vi "Example Callback.vi"() -> ()   [LabVIEW 2013]
uses:
  C:/tf/play/labview/Tinkerforge.dll
  Tinkerforge.dll
panel:
  in  "stop":bool
  in  "uid":string="63oL6P"
  in  "port":i32=4223
  in  "host":string="localhost"
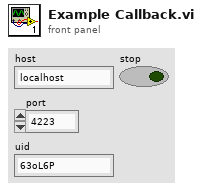
[diagram p1: front panel]
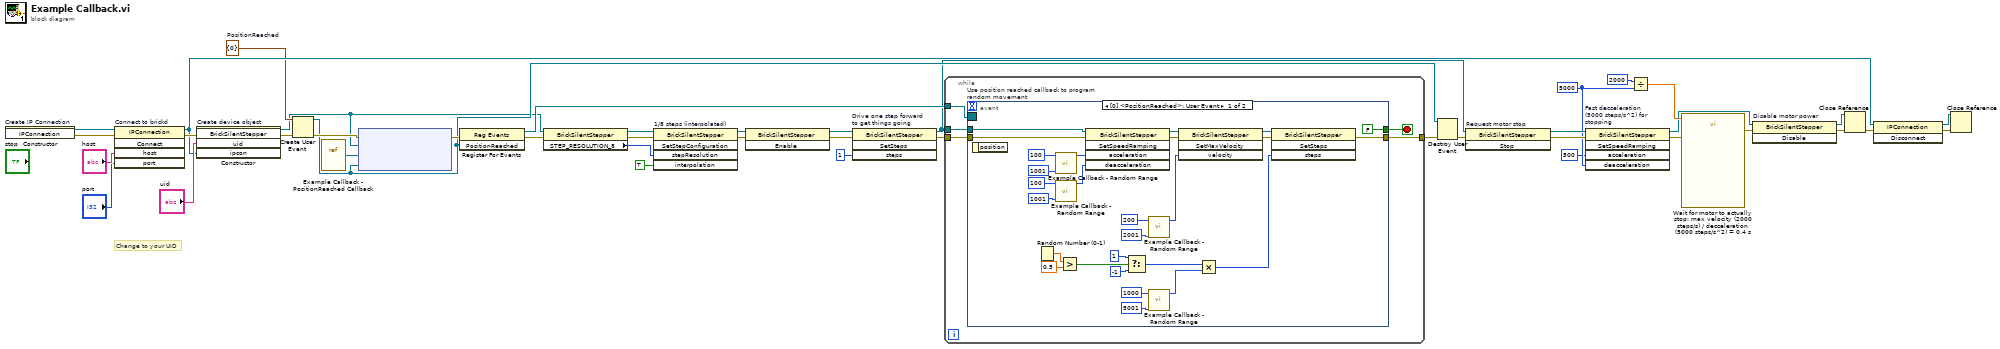
[diagram p0: block diagram]
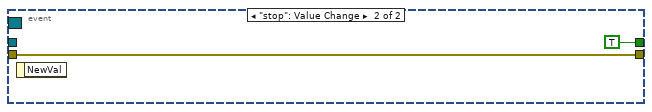
[diagram p2: hidden frame]
diagram:
  w7 = 5000 ("deacceleration")
  w29 = cluster{"position":i32} {"position"=0}  # PositionReached
  # "Change to your UID"
  n1 = constructor on="Create IP Connection" class="IPConnection"() -> (reference out=w43:refnum<k24>, error out=w23:errorcluster)  [unwired: 3 in, 1 out]
  n2 = invoke on="Connect to brickd" class="IPConnection" method="Connect"(reference=w43, error in=w23, "host"="host", "port"="port") -> (reference out=w36:refnum<k24>, error out=w39:errorcluster)  [unwired: 1 in, 3 out]
  n3 = constructor on="Create device object" class="BrickSilentStepper"(error in=w39, "uid"="uid", "ipcon"=w36) -> (reference out=w19:refnum<k24>, error out=w28:errorcluster)  [unwired: 2 in, 3 out]
  n4 = Create User Event(user event datatype=w29, error in=w28) -> (user event=w30:refnum<user-event>, error out=w34:errorcluster)
  n5 = vi-ref "Example Callback - PositionReached Callback.vi"() -> ("vi reference"=w22:refnum<vi>)
  n6 = node ("Register Event Callback")(w34, w19, w22, w30) -> (w33:errorcluster)  [unwired: 1 in, 1 out]
  n7 = register-events(error in=w33, w30) -> (reference out=w32:refnum<event-registration>, error out=w16:errorcluster)  [unwired: 1 in]
  n8 = property class="BrickSilentStepper"(reference=w19, error in=w16) -> (reference out=w18:refnum<k24>, error out=w17:errorcluster, "STEP_RESOLUTION_8"=w15:u8)
  n9 = invoke on="1/8 steps (interpolated)" class="BrickSilentStepper" method="SetStepConfiguration"(reference=w18, error in=w17, "stepResolution"=w15, "interpolation"=TRUE) -> (reference out=w20:refnum<k24>, error out=w21:errorcluster)  [unwired: 1 in, 3 out]
  n10 = invoke class="BrickSilentStepper" method="Enable"(reference=w20, error in=w21) -> (reference out=w27:refnum<k24>, error out=w26:errorcluster)  [unwired: 1 in, 1 out]
  n11 = invoke on="Drive one step forward\nto get things going" class="BrickSilentStepper" method="SetSteps"(reference=w27, error in=w26, "steps"=1) -> (reference out=w4:refnum<k24>, error out=w25:errorcluster)  [unwired: 1 in, 2 out]
  n12 = while {
    tunnel: w32 -> [w48]
    tunnel: [w47] -> w31
    tunnel: w25 -> [w46]
    tunnel: w4 -> [w45]
    stop <- w44 stop-if-true
    n13 = event "Use position reached callback to program random movement" shown="[0] <PositionReached>: User Event" {
      selector: w48 -> [_ _]
      dyn-events: _ -> [_ _]
      timeout: _ -> [_ _]
      tunnel: [w75 w76] -> w47
      tunnel: w46 -> [w71 w76]
      tunnel: w45 -> [w50 _]
      tunnel: [FALSE TRUE] -> w44
      event User Event {
        n14 = event-data() -> ()  [unwired: 1 in, 1 out]
        n15 = Random Number (0-1)() -> (number: 0 to 1=w58:dbl)
        n16 = call "Example Callback - Random Range.vi"("max"=1001, "min"=100) -> ("random"=w69:i32)  [unwired: 9 in]
        n17 = call "Example Callback - Random Range.vi"("max"=1001, "min"=100) -> ("random"=w68:i32)  [unwired: 9 in]
        n18 = Greater?(x=w58, y=0.5) -> (0:w56:bool)
        n19 = invoke class="BrickSilentStepper" method="SetSpeedRamping"(reference=w50, error in=w71, "acceleration"=w69, "deacceleration"=w68) -> (reference out=w72:refnum<k24>, error out=w70:errorcluster)  [unwired: 1 in, 3 out]
        n20 = Select(t=1, s=w56, f=-1) -> (s? t:f=w53:i32)
        n21 = call "Example Callback - Random Range.vi"("max"=2001, "min"=200) -> ("random"=w63:i32)  [unwired: 9 in]
        n22 = call "Example Callback - Random Range.vi"("max"=5001, "min"=1000) -> ("random"=w52:i32)  [unwired: 9 in]
        n23 = invoke class="BrickSilentStepper" method="SetMaxVelocity"(reference=w72, error in=w70, "velocity"=w63) -> (reference out=w74:refnum<k24>, error out=w73:errorcluster)  [unwired: 1 in, 2 out]
        n24 = Multiply(x=w53, y=w52) -> (x*y=w51:i32)
        n25 = invoke class="BrickSilentStepper" method="SetSteps"(reference=w74, error in=w73, "steps"=w51) -> (error out=w75:errorcluster)  [unwired: 1 in, 3 out]
      }
      event "stop": Value Change {
        n26 = event-data() -> ()  [unwired: 1 in, 1 out]
      }
    }
  }
  n27 = Destroy User Event(user event=w30, error in=w31) -> (error out=w5:errorcluster)
  n28 = invoke on="Request motor stop" class="BrickSilentStepper" method="Stop"(reference=w4, error in=w5) -> (reference out=w11:refnum<k24>, error out=w9:errorcluster)  [unwired: 1 in, 1 out]
  n29 = invoke on="Fast decceleration\n(5000 steps/s^2) for\nstopping" class="BrickSilentStepper" method="SetSpeedRamping"(reference=w11, error in=w9, "acceleration"=500, "deacceleration"=w7) -> (reference out=w10:refnum<k24>, error out=w8:errorcluster)  [unwired: 1 in, 3 out]
  n30 = Divide(x=2000, y=w7) -> (x/y=w12:dbl)
  n31 = call "Wait for motor to actually stop: max velocity (2000 steps/s) / decceleration (5000 steps/s^2) = 0.4 s"("error in (no error)"=w8, "Delay Time (s)"=w12) -> ("error out"=w13:errorcluster)  [unwired: 9 in]
  n32 = invoke on="Disable motor power" class="BrickSilentStepper" method="Disable"(reference=w10, error in=w13) -> (reference out=w3:refnum<k24>, error out=w2:errorcluster)  [unwired: 1 in, 1 out]
  n33 = Close Reference(reference=w3, error in (no error)=w2) -> (error out=w38:errorcluster)
  n34 = invoke class="IPConnection" method="Disconnect"(reference=w36, error in=w38) -> (reference out=w35:refnum<k24>, error out=w37:errorcluster)  [unwired: 1 in, 1 out]
  n35 = Close Reference(reference=w35, error in (no error)=w37) -> ()  [unwired: 1 out]
